vi "Start Sync.vi"(8 "error in (no error)":errorcluster, 11 "gRPC Server in":refnum<class "dcvmDPI.lvclass">) -> (0 "error out":errorcluster, 3 "gRPC Server out":refnum<class "dcvmDPI.lvclass">)   [LabVIEW 2021, in "dcvmDPI_AD7606B_server.lvlib" / "dcvmDPI.lvclass"]
uses:
  dcvmDPI.lvclass
  dcvmDPI.lvclass/dcvmDPI.ctl
  dcvmMessageQueue/controls/Message Data.ctl
  RPC Messages/dcvmDPI_IdResponse.ctl
  RPC Messages/dcvmDPI_ErrorResponse.ctl
  RPC Messages/dcvmDPI_MeasurementResponse.ctl
  RPC Messages/dcvmDPI_InitializeResponse.ctl
  RPC Messages/dcvmDPI_ConfigureResponse.ctl
  RPC Messages/dcvmDPI_InitiateResponse.ctl
  RPC Messages/dcvmDPI_AcquireResponse.ctl
  RPC Messages/dcvmDPI_CloseResponse.ctl
  dcvmMessageQueue/dcvmMessageQueue.lvlib
  dcvmDPI_AD7606B_server.lvlib
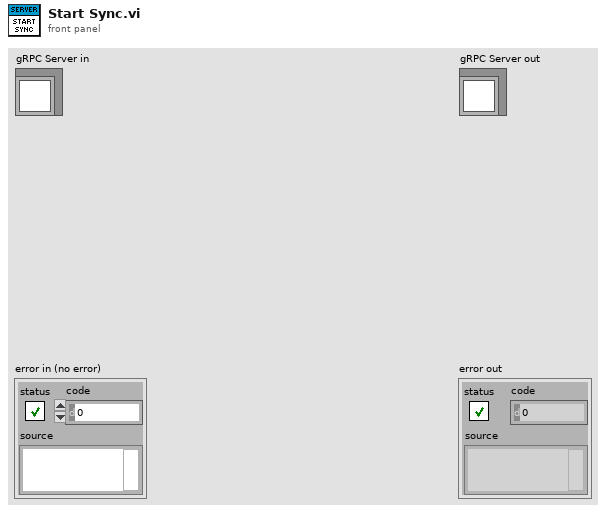
[diagram p1: front panel]
types:
  T1 = typedef "dcvmMessageQueue.lvlib/Message Queues.ctl" = cluster{"gRPC engine":refnum<queue>, "Digital engine":refnum<queue>}
  T2 = typedef "dcvmDPI_AD7606B_server.lvlib/dcvmDPI_IdResponse.ctl" = cluster{"name":string, "error":T3}
  T3 = typedef "dcvmDPI_AD7606B_server.lvlib/dcvmDPI_ErrorResponse.ctl" = cluster{"error_number":i32, "error_description":string}
  T4 = typedef "dcvmMessageQueue.lvlib/Message Data.ctl" = cluster{"Action":string, "Value":variant}
  T5 = typedef "dcvmDPI_AD7606B_server.lvlib/dcvmDPI_MeasurementResponse.ctl" = cluster{"error":T3}
  T6 = typedef "dcvmDPI_AD7606B_server.lvlib/dcvmDPI_InitializeResponse.ctl" = cluster{"error":T3}
  T7 = typedef "dcvmDPI_AD7606B_server.lvlib/dcvmDPI_ConfigureResponse.ctl" = cluster{"error":T3}
  T8 = typedef "dcvmDPI_AD7606B_server.lvlib/dcvmDPI_InitiateResponse.ctl" = cluster{"error":T3}
  T9 = typedef "dcvmDPI_AD7606B_server.lvlib/dcvmDPI_AcquireResponse.ctl" = cluster{"digital_waveform":u32[], "error":T3}
  T10 = typedef "dcvmDPI_AD7606B_server.lvlib/dcvmDPI_CloseResponse.ctl" = cluster{"error":T3}
  T11 = typedef "dcvmDPI_AD7606B_server.lvlib/dcvmDPI.lvclass/Server Internal UEs.ctl" = cluster{"dcvmDPI ID Internal UE":refnum<user-event>, "dcvmDPI ActiveMeasuresment Internal UE":refnum<user-event>, "dcvmDPI Initialize Internal UE":refnum<user-event>, "dcvmDPI Configure Internal UE":refnum<user-event>, "dcvmDPI Initiate Internal UE":refnum<user-event>, "dcvmDPI Acquire Internal UE":refnum<user-event>, "dcvmDPI Close Internal UE":refnum<user-event>}
  T12 = typedef "dcvmDPI_AD7606B_server.lvlib/dcvmDPI.lvclass/Server gRPC UEs.ctl" = cluster{"dcvmDPI ID gRPC UE":refnum<user-event>, "dcvmDPI ActiveMeasuresment gRPC UE":refnum<user-event>, "dcvmDPI Initialize gRPC UE":refnum<user-event>, "dcvmDPI Configure gRPC UE":refnum<user-event>, "dcvmDPI Initiate gRPC UE":refnum<user-event>, "dcvmDPI Acquire gRPC UE":refnum<user-event>, "dcvmDPI Close gRPC UE":refnum<user-event>}
  T13 = typedef "grpc-lvsupport-release.lvlib/grpcId.ctl" = u64
  T14 = typedef "dcvmDPI_AD7606B_server.lvlib/dcvmDPI_IdRequest.ctl" = cluster{"void":string}
  T15 = typedef "dcvmDPI_AD7606B_server.lvlib/dcvmDPI_MeasurementRequest.ctl" = cluster{"measurement":string}
  T16 = typedef "dcvmDPI_AD7606B_server.lvlib/dcvmDPI_InitializeRequest.ctl" = cluster{"device_name":string}
  T17 = typedef "dcvmDPI_AD7606B_server.lvlib/dcvmDPI_ConfigureRequest.ctl" = cluster{"digital_capture_samples":u32, "digital_capture_sample_rate":dbl, "input_channel":i32}
  T18 = typedef "dcvmDPI_AD7606B_server.lvlib/dcvmDPI_AcquireRequest.ctl" = cluster{"digital_capture_samples":u32, "timeout_ms":i32}
  T19 = typedef "dcvmDPI_AD7606B_server.lvlib/dcvmDPI_CloseRequest.ctl" = cluster{"void":string}
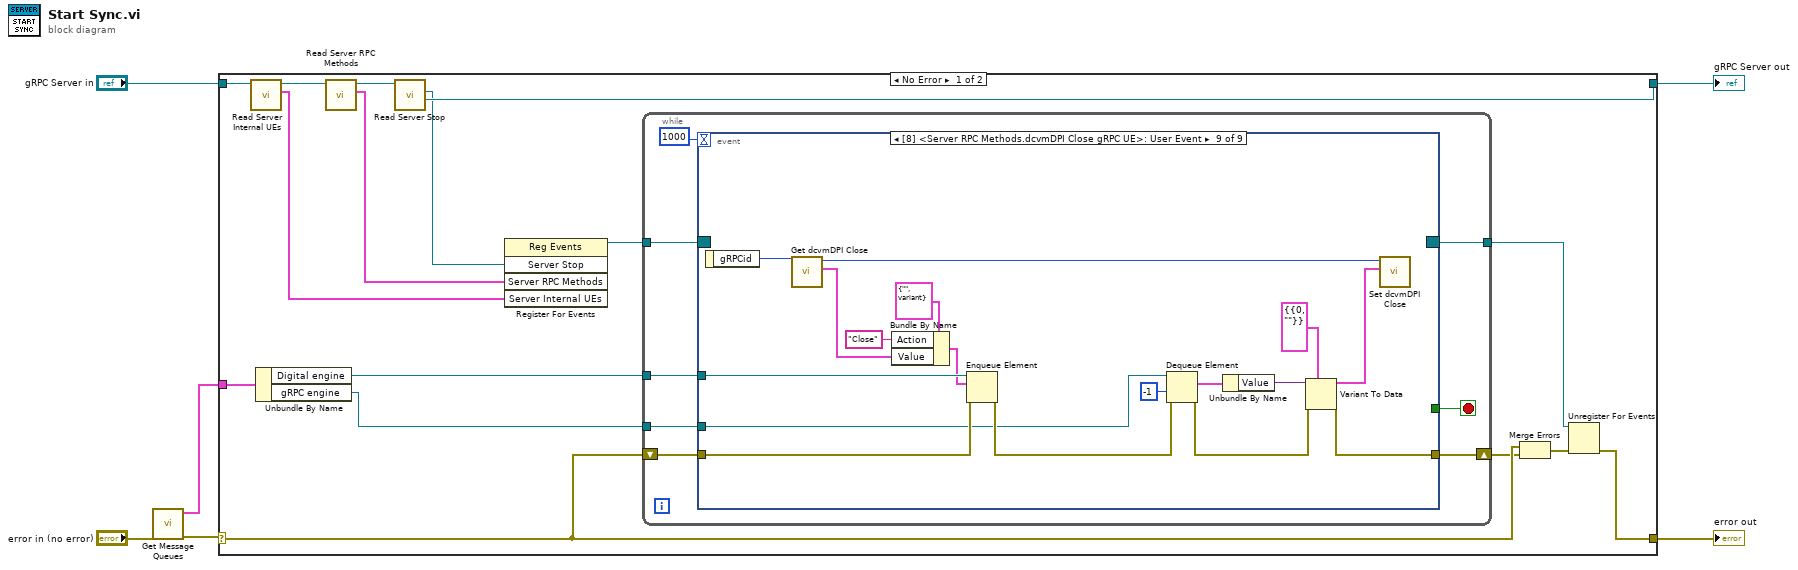
[diagram p0: block diagram]
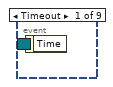
[diagram p2: hidden frame]
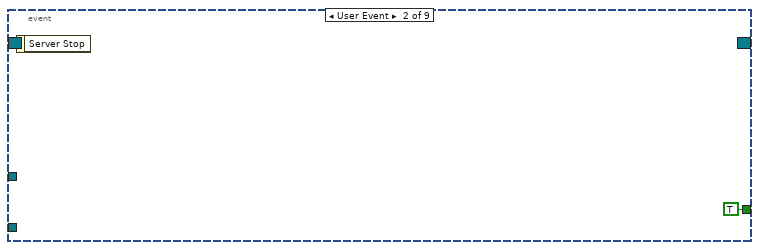
[diagram p3: hidden frame]
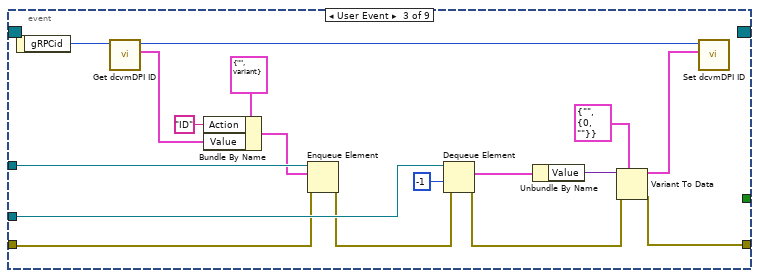
[diagram p4: hidden frame]
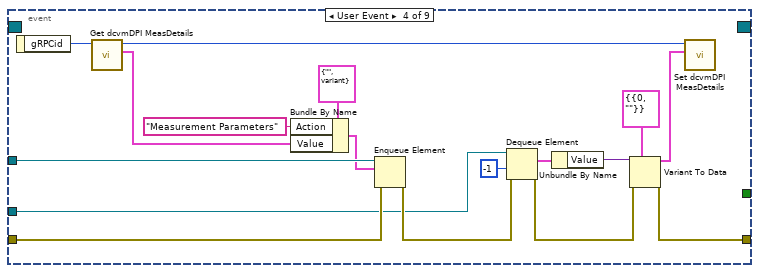
[diagram p5: hidden frame]
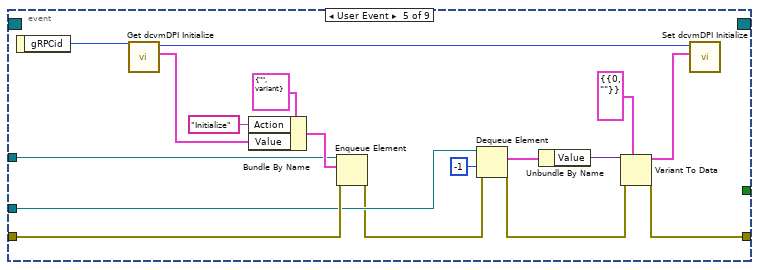
[diagram p6: hidden frame]
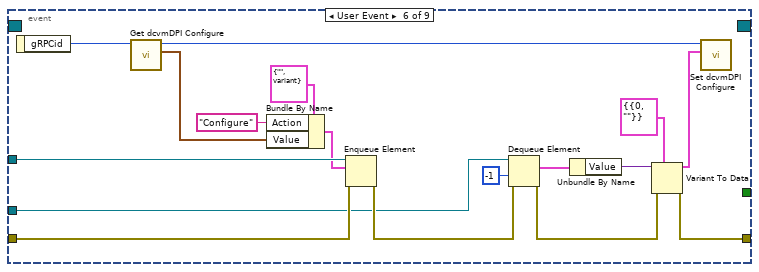
[diagram p7: hidden frame]
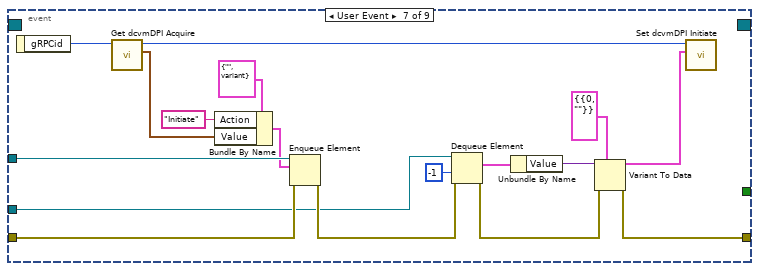
[diagram p8: hidden frame]
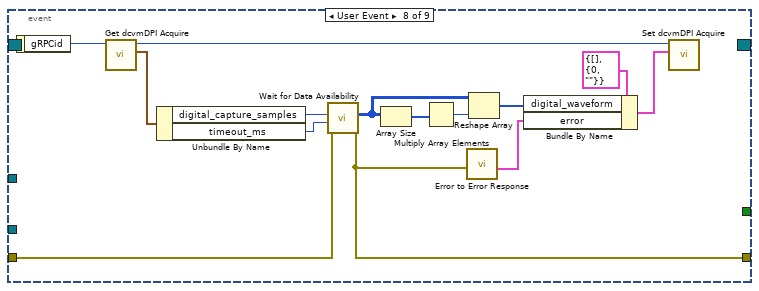
[diagram p9: hidden frame]
diagram:
  n1 = call "Get Message Queues.vi"("error in (no error)"="error in (no error)") -> ("error out"=w2:errorcluster, "AllMsgQueues QueueRef"=w1:T1)  [unwired: 8 in, 1 out]
  n2 = case shown="No Error" w2 {
    selector: w2 -> [w9 w149]
    tunnel: [w16 w149] -> w6
    tunnel: [w14 w148] -> w4
    tunnel: "gRPC Server in" -> [w22 w148]
    tunnel: w1 -> [w12 _]
    frame No Error {
      n3 = call "Read Server Internal UEs.vi"("SignalGeneratorService in"=w22) -> ("Server Internal UEs"=w20:T11, "SignalGeneratorService out"=w21:refnum<class "dcvmDPI.lvclass">)  [unwired: 8 in, 1 out]
      n4 = Unbundle By Name(w12) -> ("Digital engine"=w11:refnum<queue>, "gRPC engine"=w10:refnum<queue>)
      n5 = call "Read Server RPC Methods.vi"("SignalGeneratorService in"=w21) -> ("Server RPC Methods"=w15:T12, "SignalGeneratorService out"=w19:refnum<class "dcvmDPI.lvclass">)  [unwired: 8 in, 1 out]
      n6 = call-dynamic "Read Server Stop.vi"("iService in"=w19) -> ("Server Stop"=w13:refnum<user-event>, "iService out"=w14:refnum<class "dcvmDPI.lvclass">)  [unwired: 8 in, 1 out]
      n7 = register-events(w13, w15, w20) -> (reference out=w18:refnum<event-registration>)  [unwired: 2 in, 1 out]
      n8 = while {
        tunnel: w18 -> [w30]
        tunnel: [w28] -> w17
        tunnel: w11 -> [w26]
        tunnel: w10 -> [w25]
        shift-right: [w23] -> w8
        shift-left: w9 -> [w24]
        stop <- w29 stop-if-true
        n9 = event "RPC Methods Event Structure" shown="[8] <Server RPC Methods.dcvmDPI Close gRPC UE>: User Event" {
          selector: w30 -> [_ _ _ _ _ _ _ _ _]
          dyn-events: [_ _ _ _ _ _ _ _ _] -> w28
          timeout: 1000 -> [_ _ _ _ _ _ _ _ _]
          tunnel: [_ TRUE _ _ _ _ _ _ _] -> w29
          tunnel: w26 -> [_ _ w43 w63 w78 w98 w116 _ w147]
          tunnel: w25 -> [_ _ w41 w57 w74 w89 w111 _ w137]
          tunnel: w24 -> [_ _ w40 w59 w75 w93 w113 w126 w143]
          tunnel: [_ _ w35 w50 w66 w88 w105 w117 w138] -> w23
          event Timeout {
            n10 = event-data() -> ()  [unwired: 1 in, 1 out]
          }
          event User Event {
            n11 = event-data() -> ()  [unwired: 1 in, 1 out]
          }
          event User Event {
            n12 = event-data() -> ("gRPCid"=w48:T13)  [unwired: 1 in]
            n13 = call "Get dcvmDPI ID.vi"("gRPCid in"=w48) -> ("Message Data"=w45:T14, "gRPCid out"=w47:T13)  [unwired: 8 in, 1 out]
            n14 = Bundle By Name(cluster=T4 {"Action"="", "Value"=variant} ("Message data"), "Action"="ID", "Value"=w45) -> (w42:T4)
            n15 = Enqueue Element(queue=w43, element=w42, error in (no error)=w40) -> (error out=w38:errorcluster)  [unwired: 1 in, 2 out]
            n16 = Dequeue Element(queue=w41, timeout in ms (-1)=-1, error in (no error)=w38) -> (element=w33:T4, error out=w36:errorcluster)  [unwired: 2 out]
            n17 = Unbundle By Name(w33) -> ("Value"=w32:variant)
            n18 = Variant To Data(error in=w36, type=T2 {"name"="", "error"={"error_number"=0, "error_description"=""}} ("Message Data"), Variant=w32) -> (data=w34:T2, error out=w35:errorcluster)
            n19 = call "Set dcvmDPI ID.vi"("Message Data"=w34, "gRPCid in"=w47) -> ()  [unwired: 9 in, 1 out]
          }
          event User Event {
            n20 = event-data() -> ("gRPCid"=w65:T13)  [unwired: 1 in]
            n21 = call "Get dcvmDPI MeasDetails.vi"("gRPCid in"=w65) -> ("Message Data"=w61:T15, "gRPCid out"=w64:T13)  [unwired: 8 in, 1 out]
            n22 = Bundle By Name(cluster=T4 {"Action"="", "Value"=variant} ("Message data"), "Action"="Measurement Parameters", "Value"=w61) -> (w60:T4)
            n23 = Enqueue Element(queue=w63, element=w60, error in (no error)=w59) -> (error out=w58:errorcluster)  [unwired: 1 in, 2 out]
            n24 = Dequeue Element(queue=w57, timeout in ms (-1)=-1, error in (no error)=w58) -> (element=w55:T4, error out=w51:errorcluster)  [unwired: 2 out]
            n25 = Unbundle By Name(w55) -> ("Value"=w54:variant)
            n26 = Variant To Data(error in=w51, type=T5 {"error"={"error_number"=0, "error_description"=""}} ("Message Data"), Variant=w54) -> (data=w52:T5, error out=w50:errorcluster)
            n27 = call "Set dcvmDPI MeasDetails.vi"("Message Data"=w52, "gRPCid in"=w64) -> ()  [unwired: 9 in, 1 out]
          }
          event User Event {
            n28 = event-data() -> ("gRPCid"=w82:T13)  [unwired: 1 in]
            n29 = call "Get dcvmDPI Initialize.vi"("gRPCid in"=w82) -> ("Message Data"=w77:T16, "gRPCid out"=w81:T13)  [unwired: 8 in, 1 out]
            n30 = Bundle By Name(cluster=T4 {"Action"="", "Value"=variant} ("Message data"), "Action"="Initialize", "Value"=w77) -> (w79:T4)
            n31 = Enqueue Element(queue=w78, element=w79, error in (no error)=w75) -> (error out=w72:errorcluster)  [unwired: 1 in, 2 out]
            n32 = Dequeue Element(queue=w74, timeout in ms (-1)=-1, error in (no error)=w72) -> (element=w71:T4, error out=w67:errorcluster)  [unwired: 2 out]
            n33 = Unbundle By Name(w71) -> ("Value"=w70:variant)
            n34 = Variant To Data(error in=w67, type=T6 {"error"={"error_number"=0, "error_description"=""}} ("Message Data"), Variant=w70) -> (data=w68:T6, error out=w66:errorcluster)
            n35 = call "Set dcvmDPI Initialize.vi"("Message Data"=w68, "gRPCid in"=w81) -> ()  [unwired: 9 in, 1 out]
          }
          event User Event {
            n36 = event-data() -> ("gRPCid"=w99:T13)  [unwired: 1 in]
            n37 = call "Get dcvmDPI Configure.vi"("gRPCid in"=w99) -> ("Message Data"=w95:T17, "gRPCid out"=w85:T13)  [unwired: 8 in, 1 out]
            n38 = Bundle By Name(cluster=T4 {"Action"="", "Value"=variant} ("Message data"), "Action"="Configure", "Value"=w95) -> (w97:T4)
            n39 = Enqueue Element(queue=w98, element=w97, error in (no error)=w93) -> (error out=w92:errorcluster)  [unwired: 1 in, 2 out]
            n40 = Dequeue Element(queue=w89, timeout in ms (-1)=-1, error in (no error)=w92) -> (element=w90:T4, error out=w91:errorcluster)  [unwired: 2 out]
            n41 = Unbundle By Name(w90) -> ("Value"=w87:variant)
            n42 = Variant To Data(error in=w91, type=T7 {"error"={"error_number"=0, "error_description"=""}} ("Message Data"), Variant=w87) -> (data=w83:T7, error out=w88:errorcluster)
            n43 = call "Set dcvmDPI Configure.vi"("Message Data"=w83, "gRPCid in"=w85) -> ()  [unwired: 9 in, 1 out]
          }
          event User Event {
            n44 = event-data() -> ("gRPCid"=w104:T13)  [unwired: 1 in]
            n45 = call "Get dcvmDPI Acquire.vi"("gRPCid in"=w104) -> ("Message Data"=w103:T18, "gRPCid out"=w102:T13)  [unwired: 8 in, 1 out]
            n46 = Bundle By Name(cluster=T4 {"Action"="", "Value"=variant} ("Message data"), "Action"="Initiate", "Value"=w103) -> (w114:T4)
            n47 = Enqueue Element(queue=w116, element=w114, error in (no error)=w113) -> (error out=w112:errorcluster)  [unwired: 1 in, 2 out]
            n48 = Dequeue Element(queue=w111, timeout in ms (-1)=-1, error in (no error)=w112) -> (element=w108:T4, error out=w106:errorcluster)  [unwired: 2 out]
            n49 = Unbundle By Name(w108) -> ("Value"=w107:variant)
            n50 = Variant To Data(error in=w106, type=T8 {"error"={"error_number"=0, "error_description"=""}} ("data"), Variant=w107) -> (data=w101:T8, error out=w105:errorcluster)
            n51 = call "Set dcvmDPI Initiate.vi"("Message Data"=w101, "gRPCid in"=w102) -> ()  [unwired: 9 in, 1 out]
          }
          event User Event {
            n52 = event-data() -> ("gRPCid"=w130:T13)  [unwired: 1 in]
            n53 = call "Get dcvmDPI Acquire.vi"("gRPCid in"=w130) -> ("Message Data"=w129:T18, "gRPCid out"=w122:T13)  [unwired: 8 in, 1 out]
            n54 = Unbundle By Name(w129) -> ("digital_capture_samples"=w128:u32, "timeout_ms"=w127:i32)
            n55 = call "Wait for Data Availability.vi"("error in"=w126, "Time out"=w127, "Samples to read"=w128) -> ("error out"=w117:errorcluster, "Data out"=w124:u32[][])  [unwired: 7 in]
            n56 = Array Size(array=w124) -> (size(s)=w125:i32[])
            n57 = Multiply Array Elements(1:w125) -> (0:w123:i32)
            n58 = call "Error to Error Response.vi"("error in (no error)"=w117) -> ("error response"=w119:T3)  [unwired: 10 in]
            n59 = Reshape Array(w124, w123) -> (w120:u32[])
            n60 = Bundle By Name(cluster=T9 {"digital_waveform"=[], "error"={"error_number"=0, "error_description"=""}} ("Message Data"), "digital_waveform"=w120, "error"=w119) -> (w118:T9)
            n61 = call "Set dcvmDPI Acquire.vi"("Message Data"=w118, "gRPCid in"=w122) -> ()  [unwired: 9 in, 1 out]
          }
          event User Event {
            n62 = event-data() -> ("gRPCid"=w135:T13)  [unwired: 1 in]
            n63 = call "Get dcvmDPI Close.vi"("gRPCid in"=w135) -> ("Message Data"=w134:T19, "gRPCid out"=w133:T13)  [unwired: 8 in, 1 out]
            n64 = Bundle By Name(cluster=T4 {"Action"="", "Value"=variant} ("Message data"), "Action"="Close", "Value"=w134) -> (w145:T4)
            n65 = Enqueue Element(queue=w147, element=w145, error in (no error)=w143) -> (error out=w142:errorcluster)  [unwired: 1 in, 2 out]
            n66 = Dequeue Element(queue=w137, timeout in ms (-1)=-1, error in (no error)=w142) -> (element=w140:T4, error out=w141:errorcluster)  [unwired: 2 out]
            n67 = Unbundle By Name(w140) -> ("Value"=w139:variant)
            n68 = Variant To Data(error in=w141, type=T10 {"error"={"error_number"=0, "error_description"=""}} ("data"), Variant=w139) -> (data=w132:T10, error out=w138:errorcluster)
            n69 = call "Set dcvmDPI Close.vi"("Message Data"=w132, "gRPCid in"=w133) -> ()  [unwired: 9 in, 1 out]
          }
        }
      }
      n70 = Merge Errors(w9, w8) -> (w7:errorcluster)
      n71 = Unregister For Events(event registration refnum=w17, error in=w7) -> (error out=w16:errorcluster)
    }
    frame Error {
    }
  }
  "error out" <- w6
  "gRPC Server out" <- w4
